vi "Init.vi"(8 "error in (no error)":errorcluster, 10 "Godot":refnum<class "GodotServer.lvclass">) -> (0 "error out":errorcluster, 3 "FormulaG API out":refnum<class "FormulaG API.lvclass">)   [LabVIEW 2024, in "FormulaG.lvlib" / "FormulaG API.lvclass"]
uses:
  FormulaG API.lvclass
  <vilib>/IlluminatedG/IG GodotServer/GodotLV/GodotServer/GodotServer.lvclass
  FormulaG API.lvclass/FormulaG API.ctl
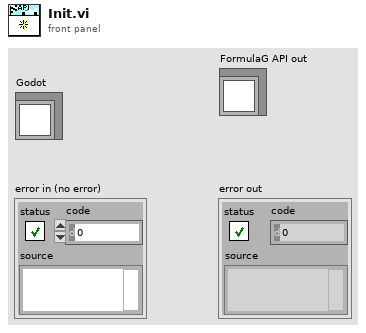
[diagram p1: front panel]
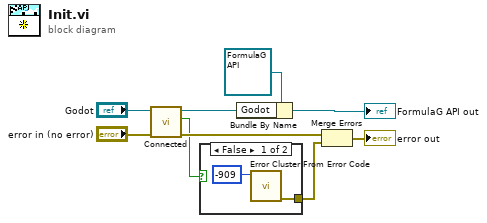
[diagram p0: block diagram]
diagram:
  n1 = call <vilib>:"Connected.vi"("error in (no error)"="error in (no error)", "GodotServer in"="Godot") -> ("error out"=w6:errorcluster, "Connected"=w3:bool, "GodotServer out"=w4:refnum<class "GodotServer.lvclass">)  [unwired: 7 in]
  n2 = case shown="False" w3 {
    tunnel: [w10 _] -> w1
    frame False {
      n3 = call <vilib>:"Error Cluster From Error Code.vi"("error code (0)"=-909) -> ("error out"=w10:errorcluster)  [unwired: 8 in]
    }
    frame True {
    }
  }
  n4 = Bundle By Name(cluster=refnum<class "FormulaG API.lvclass"> refnum ("FormulaG API in"), "Godot"=w4) -> (→"FormulaG API out":refnum<class "FormulaG API.lvclass">)
  n5 = Merge Errors(w6, w1) -> (→"error out":errorcluster)
